vi "Basic-Final-Project.vi"() -> ()   [LabVIEW 2018]
panel:
  in  "Stop Button":bool
  in  "Calculate":bool
  in  "Conversion Selector":bool
  out "Output Temperature":dbl=32.0
  in  "Input Temperature":dbl
  # "C -> F"
  # "F -> C"
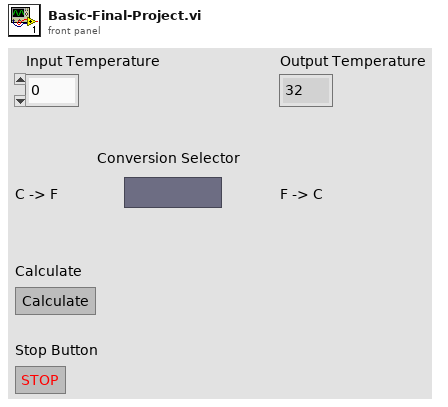
[diagram p1: front panel]
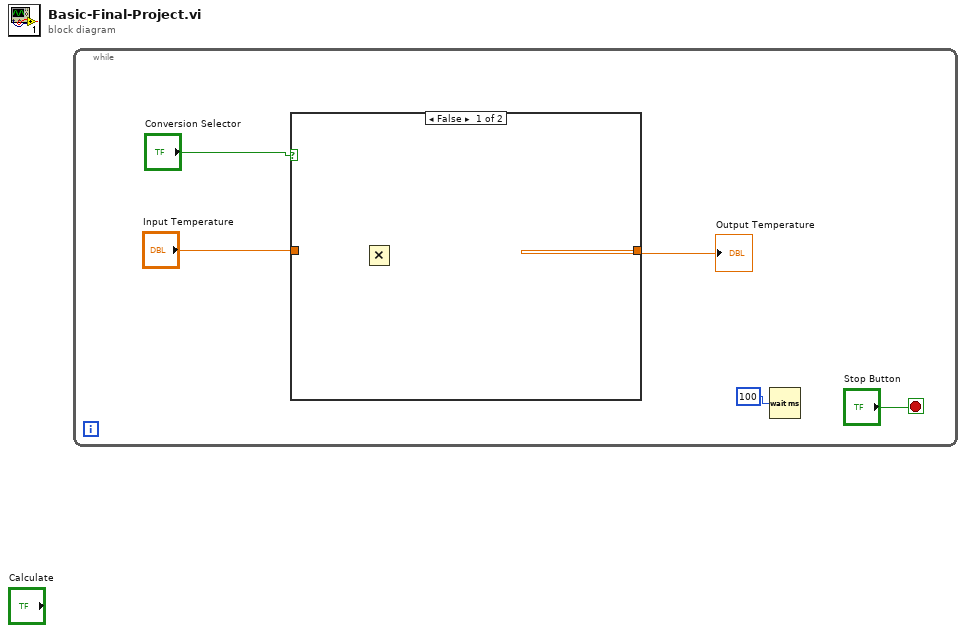
[diagram p0: block diagram]
diagram:
  n1 = while {
    stop <- "Stop Button" stop-if-true
    n2 = case shown="False" "Conversion Selector" {
      tunnel: "Input Temperature" -> [_ w6]
      tunnel: [_ w6] -> w1
      frame False {
        n3 = Multiply() -> ()  [unwired: 2 in, 1 out]
      }
      frame True {
      }
    }
    "Output Temperature" <- w1
    n4 = Wait (ms)(milliseconds to wait=u32 100) -> ()  [unwired: 1 out]
  }
